vi "SetCursorPos.vi"(8 "error in":errorcluster, 11 "Position":cluster{"X":i32, "Y":i32}) -> (0 "error out":errorcluster)   [LabVIEW 2015]
uses:
  user32.dll
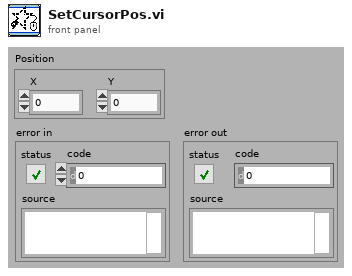
[diagram p1: front panel]
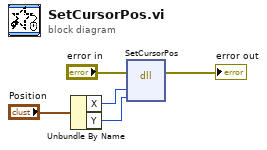
[diagram p0: block diagram]
diagram:
  n1 = Unbundle By Name("Position") -> ("X"=w5:i32, "Y"=w4:i32)
  n2 = dll-call lib="User32.dll" fn="SetCursorPos"(error in="error in", "dx"=w5, "dy"=w4) -> (error out=→"error out":errorcluster)  [unwired: 5 in, 1 out]
